vi "SetMode.vi"(8 "error in (no error)":errorcluster, 11 "Laser Diode Controller in":refnum<class "KLD101.lvclass">) -> (0 "error out":errorcluster, 3 "Laser Diode Controller out":refnum<class "KLD101.lvclass">)   [LabVIEW 2016, in "Laser Diode Controller.lvlib" / "KLD101.lvclass"]
uses:
  KLD101.lvclass
  KLD101.lvclass/KLD101.ctl
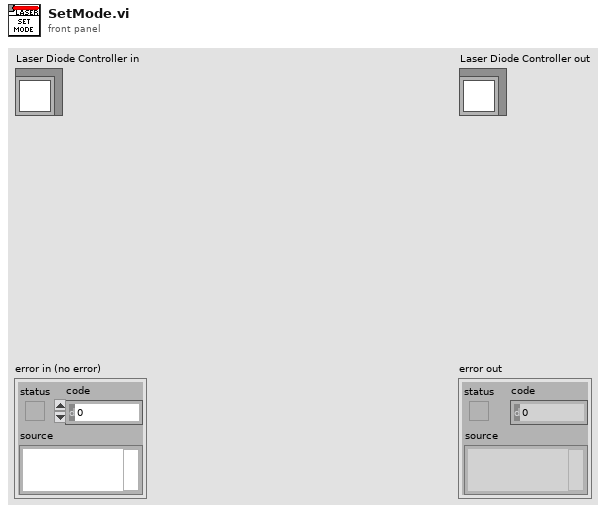
[diagram p1: front panel]
types:
  T1 = typedef "Configuration.lvlib/Config Data.lvclass/LaserMode.ctl" = enum16{"Constant Power", "Constant Current"}
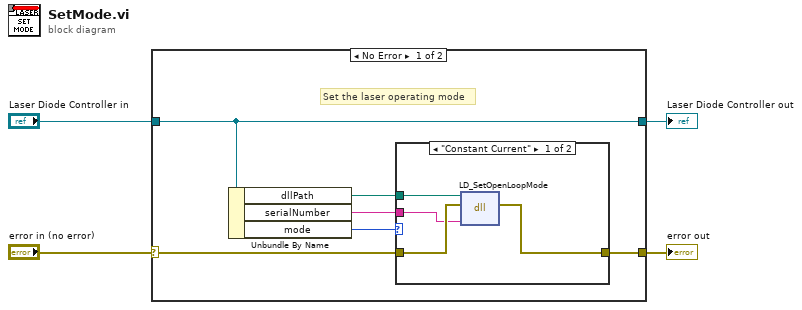
[diagram p0: block diagram]
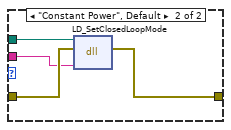
[diagram p2: hidden frame]
diagram:
  n1 = case shown="No Error" "error in (no error)" {
    selector: "error in (no error)" -> [w9 w20]
    tunnel: [w8 w20] -> w3
    tunnel: [w10 w19] -> w1
    tunnel: "Laser Diode Controller in" -> [w10 w19]
    frame No Error {
      # "Set the laser operating mode"
      n2 = Unbundle By Name(w10) -> ("dllPath"=w5:path, "serialNumber"=w7:string, "mode"=w6:T1)
      n3 = case shown="\"Constant Current\"" w6 {
        tunnel: w9 -> [w14 w18]
        tunnel: [w13 w17] -> w8
        tunnel: w7 -> [w12 w16]
        tunnel: w5 -> [w11 w15]
        frame "Constant Current" {
          n4 = dll-call lib="C:/IDEXX Software/Collimation/data/Thorlabs.MotionControl.KCube.LaserDiode.dll" fn="LD_SetOpenLoopMode"(path in=w11, error in=w14, "serialNumber"=w12) -> (error out=w13:errorcluster)  [unwired: 3 in, 1 out]
        }
        frame "Constant Power", Default {
          n5 = dll-call lib="C:/IDEXX Software/Collimation/data/Thorlabs.MotionControl.KCube.LaserDiode.dll" fn="LD_SetClosedLoopMode"(path in=w15, error in=w18, "serialNumber"=w16) -> (error out=w17:errorcluster)  [unwired: 3 in, 1 out]
        }
      }
    }
    frame Error {
    }
  }
  "error out" <- w3
  "Laser Diode Controller out" <- w1
